vi "Pulse - Set Init and Trans Curr.vi"(8 "error in (no error)":errorcluster, 10 "Trigger Settings":T1, 11 "3300 in":refnum<class "3300.lvclass">) -> (0 "error out":errorcluster, 3 "3300 out":refnum<class "3300.lvclass">)   [LabVIEW 2019, in "3300.lvlib" / "3300.lvclass"]
uses:
  Library/3300.lvclass
  builds/Instruments/Electronic Load.lvlibp/Custom Controls/Trigger Settings.ctl
  builds/Instruments/Electronic Load.lvlibp/Custom Controls/E-Load Mode.ctl
  Library/3300.lvclass/3300.ctl
  Accessors/Read Local Resource.vi
  Accessors/Write Local Resource.vi
  <instrlib>/Agilent N330X Series/Agilent N330X Series.lvlib
  builds/Instruments/Electronic Load.lvlibp/Library/Electronic Load.lvclass
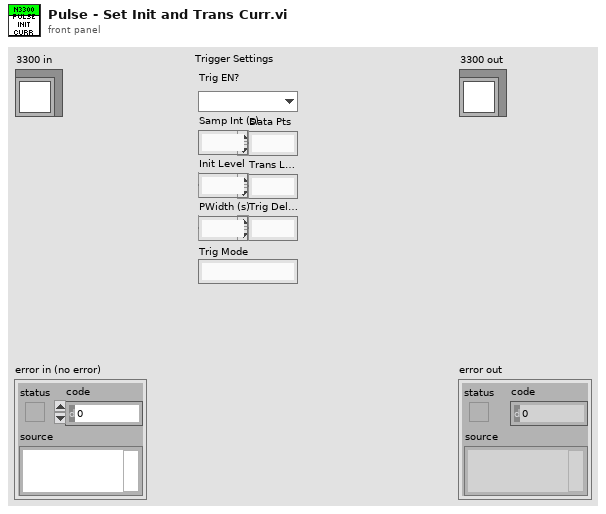
[diagram p1: front panel]
types:
  T1 = typedef "Electronic Load.lvlibp/Electronic Load.lvclass/Trigger Settings.ctl" = cluster{"Mode":T2, "Initial":dbl, "Transient":dbl, "Interval":dbl, "Width":dbl, "Delay":dbl, "Data Pts":i32, "Slew Rate":dbl}
  T2 = typedef "Electronic Load.lvlibp/Electronic Load.lvclass/E-Load Mode.ctl" = enum16{"Current", "Resistance", "Voltage"}
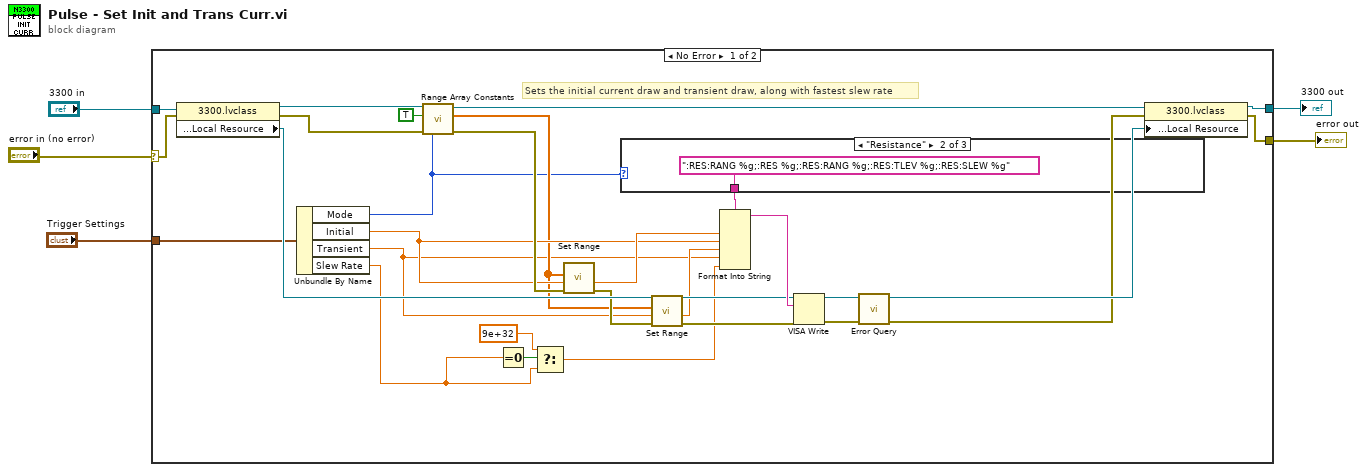
[diagram p0: block diagram]
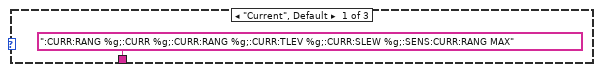
[diagram p2: hidden frame]
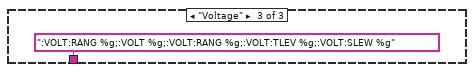
[diagram p3: hidden frame]
diagram:
  n1 = case shown="No Error" "error in (no error)" {
    selector: "error in (no error)" -> [w33 w39]
    tunnel: [w29 w39] -> w3
    tunnel: [w32 w38] -> w4
    tunnel: "3300 in" -> [w27 w38]
    tunnel: "Trigger Settings" -> [w12 _]
    frame No Error {
      # "Sets the initial current draw and transient draw, along with fastest slew rate"
      n2 = property class="3300.lvclass"(reference=w27, error in=w33) -> (reference out=w24:refnum<class "3300.lvclass">, error out=w22:errorcluster, "Private:Accessors:Local Resource"=w28:refnum<visa-resource-name>)
      n3 = Unbundle By Name(w12) -> ("Mode"=w7:T2, "Initial"=w19:dbl, "Transient"=w13:dbl, "Slew Rate"=w9:dbl)
      n4 = call "Range Array Constants.vi"("Triggered Mode"=w7, "error in (no error)"=w22, "Triggered?"=TRUE, "3300 in"=w24) -> ("error out"=w21:errorcluster, "Range Array"=w16:dbl[], "3300 out"=w23:refnum<class "3300.lvclass">)  [unwired: 5 in]
      n5 = Equal To 0?(x=w9) -> (x = 0?=w11:bool)
      n6 = Select(t=9e+32, s=w11, f=w9) -> (s? t:f=w8:dbl)
      n7 = call "Set Range.vi"("error in (no error)"=w21, "Input Level"=w19, "Range Array"=w16) -> ("error out"=w17:errorcluster, "Range"=w20:dbl)  [unwired: 6 in, 1 out]
      n8 = case shown="\"Resistance\"" w7 {
        tunnel: [":CURR:RANG %g;:CURR %g;:CURR:RANG %g;:CURR:TLEV %g;:CURR:SLEW %g;:SENS:CURR:RANG MAX" ("string (\"\")") ":RES:RANG %g;:RES %g;:RES:RANG %g;:RES:TLEV %g;:RES:SLEW %g" ("string (\"\")") ":VOLT:RANG %g;:VOLT %g;:VOLT:RANG %g;:VOLT:TLEV %g;:VOLT:SLEW %g" ("string (\"\")")] -> w6
        frame "Current", Default {
        }
        frame "Resistance" {
        }
        frame "Voltage" {
        }
      }
      n9 = call "Set Range.vi"("error in (no error)"=w17, "Input Level"=w13, "Range Array"=w16) -> ("error out"=w15:errorcluster, "Range"=w14:dbl)  [unwired: 6 in, 1 out]
      n10 = Format Into String(format string=w6, w20, w19, w14, w13, w8) -> (resulting string=w34:string)  [unwired: 2 in, 1 out]
      n11 = VISA Write(VISA resource name=w28, write buffer=w34, error in (no error)=w15) -> (VISA resource name out=w26:refnum<visa-resource-name>, error out=w25:errorcluster)  [unwired: 1 out]
      n12 = call <instrlib>:"Error Query.vi"("error in (no error)"=w25, "VISA resource name"=w26) -> ("error out"=w30:errorcluster, "VISA resource name out"=w31:refnum<visa-resource-name>)  [unwired: 6 in, 2 out]
      n13 = property class="3300.lvclass"(reference=w23, error in=w30, "Private:Accessors:Local Resource"=w31) -> (reference out=w32:refnum<class "3300.lvclass">, error out=w29:errorcluster)
    }
    frame Error {
    }
  }
  "error out" <- w3
  "3300 out" <- w4
